vi "2bfactorial.vi"() -> ()   [LabVIEW 2013]
panel:
  out "output":dbl
  in  "input":dbl
  in  "const":dbl
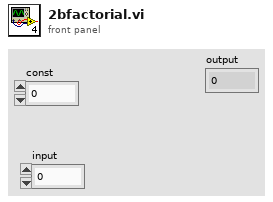
[diagram p1: front panel]
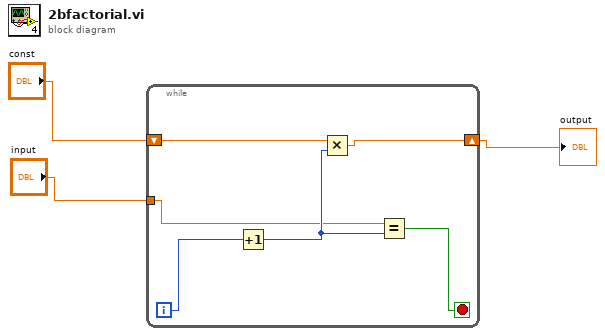
[diagram p0: block diagram]
diagram:
  n1 = while {
    tunnel: "input" -> [w6]
    shift-right: [w4] -> w1
    shift-left: "const" -> [w5]
    i -> [w8]
    stop <- w9 stop-if-true
    n2 = Increment(x=w8) -> (x+1=w7:i32)
    n3 = Multiply(x=w5, y=w7) -> (x*y=w4:dbl)
    n4 = Equal?(x=w6, y=w7) -> (x = y?=w9:bool)
  }
  "output" <- w1
